vi "String length.vi"() -> ()   [LabVIEW 2020]
panel:
  out "Batch Length":i32
  out "Actual Bitrate kHz 2":i32=1000
  out "dup Cheetah Handle":i32
  out "Total Shifted Out":i32
  out "Actual Bitrate kHz":i32=1000
  out "error out":errorcluster
  in  "Rds per Sec":dbl=2000.0 max=2000000000.0
  out "SDO":u64[](array[numeric]) format="%x"
  in  "SCLK (kHz)":i32=2000 min=0
  out "Cheetah Handle":i32
  out "if false":string
  out "Result of comparission":string
  out "Length in bytes":i32
  out "SDI":u64[](array[numeric]) format="%.0x"
  out "Array":string[](array[string])
  in  "String":string
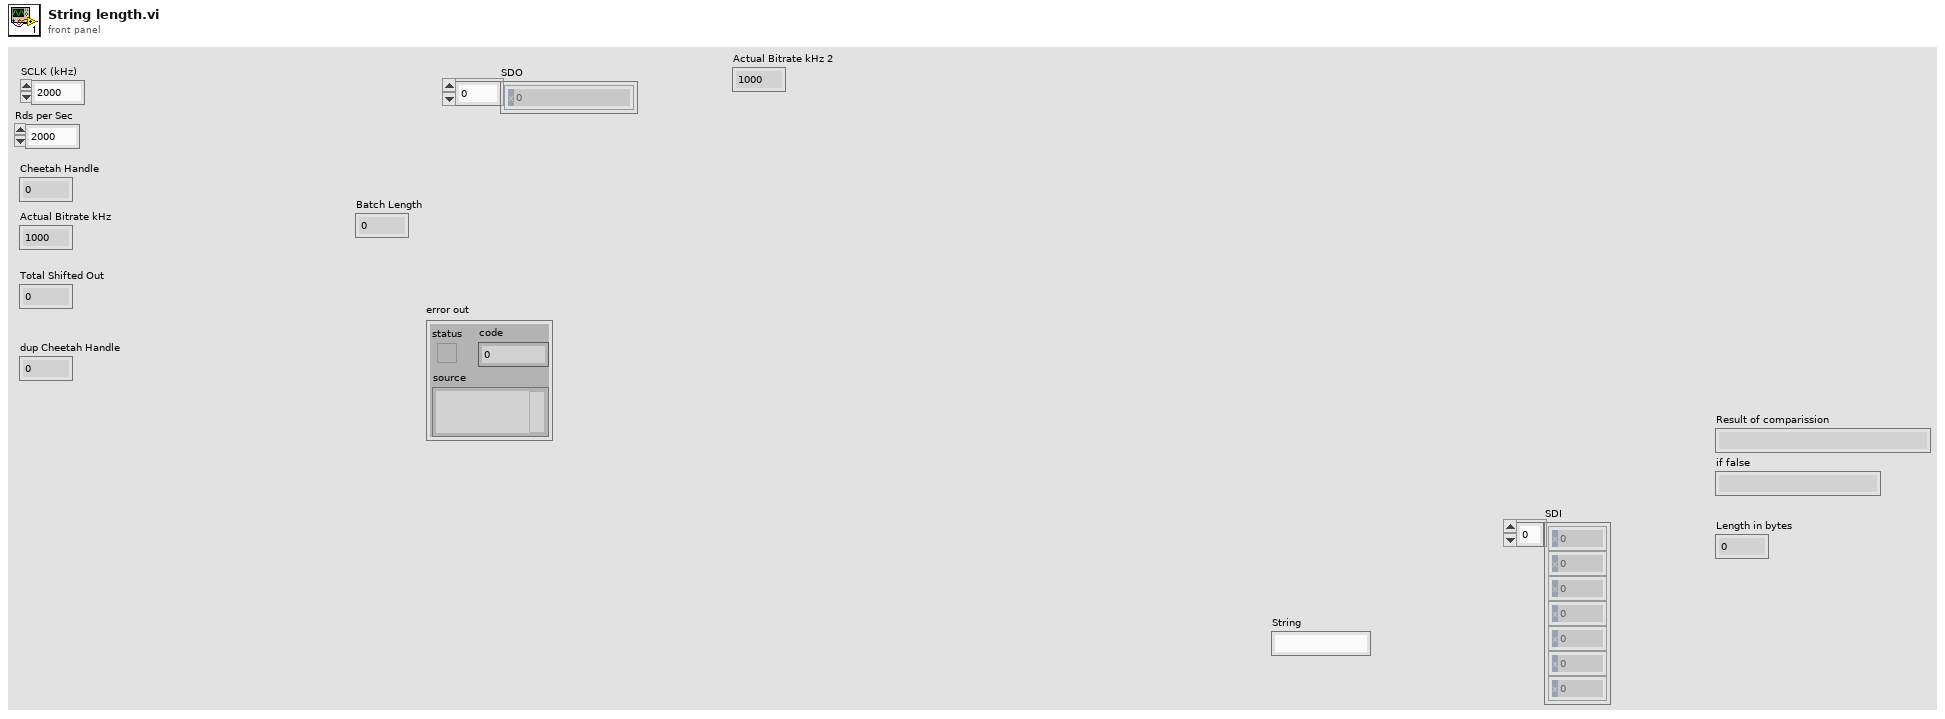
[diagram p1: front panel]
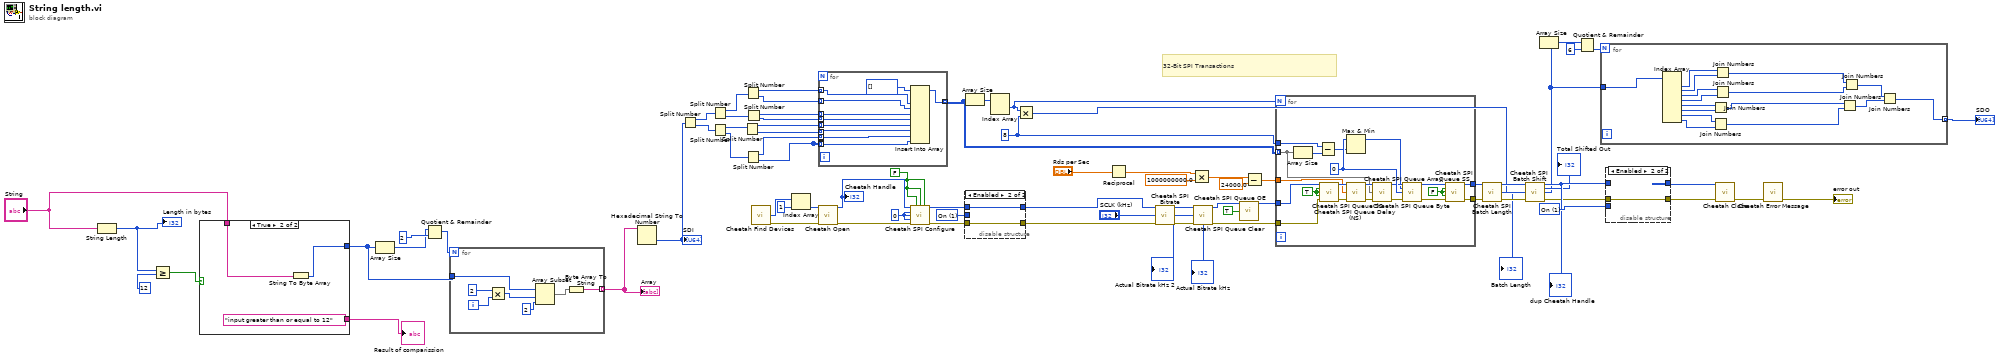
[diagram p0: block diagram]
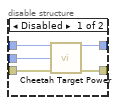
[diagram p2: hidden frame]
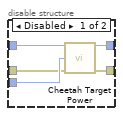
[diagram p3: hidden frame]
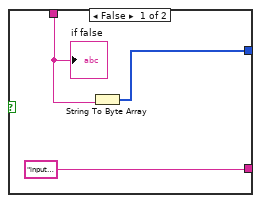
[diagram p4: hidden frame]
diagram:
  w20 = 8 ("y")
  w45 = u16 1 items=["Off", "On", "Query"] ("Requested Configuration (2: Query)")
  w46 = u16 1 items=["Off", "On", "Query"] ("Requested Configuration (2: Query)")
  w61 = FALSE
  w63 = 0
  # "32-Bit SPI Transactions"
  n1 = String Length(string="String") -> (length=w68:i32)
  "Length in bytes" <- w68
  n2 = Greater Or Equal?(x=w68, y=12) -> (x >= y?=w72:bool)
  n3 = case shown="True" w72 {
    tunnel: [w76 w81] -> w71
    tunnel: "String" -> [w77 w80]
    tunnel: ["input less than 12" "input greater than or equal to 12"] -> w69
    frame False {
      n4 = String To Byte Array(string=w77) -> (unsigned byte array=w76:u8[])
      "if false" <- w77
    }
    frame True {
      n5 = String To Byte Array(string=w80) -> (unsigned byte array=w81:u8[])
    }
  }
  "Result of comparission" <- w69
  n6 = Array Size(array=w71) -> (size(s)=w66:i32)
  n7 = Quotient & Remainder(x=w66, y=2) -> (floor(x/y)=w75:i32)  [unwired: 1 out]
  n8 = for {
    N: w75 -> [_]
    tunnel: w71 -> [w88]
    tunnel: [w85] -> w74 mode=indexing
    i -> [w83]
    n9 = Multiply(x=2 ("y"), y=w83) -> (x*y=w87:i32)
    n10 = Array Subset(array=w88, index=w87, length=2) -> (w84:u8[])
    n11 = Byte Array To String(unsigned byte array=w84) -> (string=w85:string)
  }
  "Array" <- w74
  n12 = Hexadecimal String To Number(string=w74) -> (number=w1:u32[])  [unwired: 2 in, 1 out]
  "SDI" <- w1
  n13 = Split Number(x=w1) -> (hi(x)=w31:u16[], lo(x)=w30:u16[])
  n14 = Split Number(x=w31) -> (hi(x)=w8:u8[], lo(x)=w7:u8[])
  n15 = Split Number(x=w30) -> (hi(x)=w10:u8[], lo(x)=w9:u8[])
  n16 = Split Number(x=w10) -> (hi(x)=w14:u8[], lo(x)=w13:u8[])
  n17 = Split Number(x=w8) -> (hi(x)=w6:u8[], lo(x)=w5:u8[])
  n18 = Split Number(x=w9) -> (hi(x)=w12:u8[], lo(x)=w11:u8[])
  n19 = Split Number(x=w7) -> (hi(x)=w4:u8[], lo(x)=w3:u8[])
  n20 = call <instrlib>:"Cheetah Find Devices.vi"() -> ("Ports"=w64:u16[], "error out"=w60:errorcluster)  [unwired: 13 in, 1 out]
  n21 = Index Array(array=w64, index=1) -> (element=w52:u16)
  n22 = for {
    tunnel: w14 -> [w98] mode=indexing
    tunnel: [w97] -> w29 mode=indexing
    tunnel: w12 -> [w95] mode=indexing
    tunnel: w11 -> [_] mode=indexing
    tunnel: w11 -> [w94] mode=indexing
    tunnel: w13 -> [w93] mode=indexing
    tunnel: w6 -> [w92] mode=indexing
    tunnel: w5 -> [w91] mode=indexing
    tunnel: w4 -> [w90] mode=indexing
    tunnel: w3 -> [w89] mode=indexing
    n23 = Insert Into Array(array=u8[] [], new element #1=w92, new element #2=w91, new element #3=w90, new element #4=w89, new element #5=w98, new element #6=w93, new element #7=w95, new element #8=w94) -> (w97:u8[])  [unwired: 1 in]
  }
  n24 = call <instrlib>:"Cheetah Open.vi"("Port Number (0)"=w52, "error in (no error)"=w60) -> ("Cheetah Handle"=w57:i32, "error out"=w59:errorcluster)  [unwired: 12 in]
  "Cheetah Handle" <- w57
  n25 = call <instrlib>:"Cheetah SPI Configure.vi"("Cheetah Handle"=w57, "SS0 Active High? (False)"=w61, "SS1 Active High? (False)"=w61, "SS2 Active High? (False)"=w61, "Polarity (0: Rising/Falling)"=w63, "Phase (0: Sample/Setup)"=w63, "Bitorder (0: MSB)"=w63, "error in (no error)"=w59) -> ("dup Cheetah Handle"=w56:i32, "error out"=w58:errorcluster)  [unwired: 6 in]
  n26 = disable-structure shown="Enabled" {
    disable-tunnel: w58 -> [w103 w104]
    disable-tunnel: w56 -> [w102 w105]
    disable-tunnel: [w101 w104] -> w55
    disable-tunnel: [w100 w105] -> w53
    disable-tunnel: w45 -> [w99 _]
    frame Disabled {
      n27 = call <instrlib>:"Cheetah Target Power.vi"("Cheetah Handle"=w102, "Requested Configuration (2: Query)"=w99, "error in (no error)"=w103) -> ("dup Cheetah Handle"=w100:i32, "error out"=w101:errorcluster)  [unwired: 10 in, 1 out]
    }
    frame Enabled {
    }
  }
  n28 = Array Size(array=w29) -> (size(s)=w44:i32[])
  n29 = Index Array(array=w44) -> (element #1=w16:i32)  [unwired: 2 in, 1 out]
  n30 = Multiply(x=w16, y=w20) -> (x*y=w15:i32)
  n31 = Reciprocal(x="Rds per Sec") -> (1/x=w22:dbl)
  n32 = call <instrlib>:"Cheetah SPI Bitrate.vi"("Cheetah Handle"=w53, "Requested Bitrate kHz (1000)"="SCLK (kHz)", "error in (no error)"=w55) -> ("dup Cheetah Handle"=w51:i32, "Actual Bitrate kHz"=→"Actual Bitrate kHz" →"Actual Bitrate kHz 2":i32, "error out"=w50:errorcluster)  [unwired: 10 in]
  n33 = Multiply(x=w22, y=1000000000.0) -> (x*y=w25:dbl)
  n34 = call <instrlib>:"Cheetah SPI Queue Clear.vi"("Cheetah Handle"=w51, "error in (no error)"=w50) -> ("dup Cheetah Handle"=w43:i32, "error out"=w62:errorcluster)  [unwired: 12 in]
  n35 = call <instrlib>:"Cheetah SPI Queue OE.vi"("Cheetah Handle"=w43, "Output Enable (on)"=TRUE) -> ("dup Cheetah Handle"=w42:i32)  [unwired: 12 in, 1 out]
  n36 = Subtract(x=w25, y=24000.0) -> (x-y=w23:dbl)
  n37 = for {
    N: w16 -> [_]
    tunnel: w62 -> [w112]
    tunnel: w42 -> [w113]
    tunnel: w29 -> [w114] mode=indexing
    tunnel: [w111] -> w40
    tunnel: [w110] -> w39
    tunnel: w23 -> [w107]
    tunnel: w20 -> [w108]
    w118 = FALSE
    w121 = 0
    w109 = TRUE
    n38 = Array Size(array=w114) -> (size(s)=w115:i32)
    n39 = Subtract(x=w108, y=w115) -> (x-y=w119:i32)
    n40 = call <instrlib>:"Cheetah SPI Queue SS.vi"("Cheetah Handle"=w113, "SS0 Assert? (True)"=w109, "SS1 Assert? (True)"=w109, "SS2 Assert? (True)"=w109, "error in (no error)"=w112) -> ("dup Cheetah Handle"=w126:i32, "error out"=w125:errorcluster)  [unwired: 9 in]
    n41 = Max & Min(x=w121, y=w119) -> (max(x,y)=w106:i32)  [unwired: 1 out]
    n42 = call <instrlib>:"Cheetah SPI Queue Delay (NS).vi"("Cheetah Handle"=w126, "Delay NS (1000)"=w107, "error in (no error)"=w125) -> ("dup Cheetah Handle"=w124:i32, "error out"=w123:errorcluster)  [unwired: 10 in, 1 out]
    n43 = call <instrlib>:"Cheetah SPI Queue Array.vi"("Cheetah Handle"=w124, "Data Out (none)"=w114, "error in (no error)"=w123) -> ("dup Cheetah Handle"=w120:i32, "error out"=w122:errorcluster)  [unwired: 11 in]
    n44 = call <instrlib>:"Cheetah SPI Queue Byte.vi"("Cheetah Handle"=w120, "Byte Count (1)"=w106, "Byte Value (0x00)"=w121, "error in (no error)"=w122) -> ("dup Cheetah Handle"=w117:i32, "error out"=w116:errorcluster)  [unwired: 10 in]
    n45 = call <instrlib>:"Cheetah SPI Queue SS.vi"("Cheetah Handle"=w117, "SS0 Assert? (True)"=w118, "SS1 Assert? (True)"=w118, "SS2 Assert? (True)"=w118, "error in (no error)"=w116) -> ("dup Cheetah Handle"=w110:i32, "error out"=w111:errorcluster)  [unwired: 9 in]
  }
  n46 = call <instrlib>:"Cheetah SPI Batch Length.vi"("Cheetah Handle"=w39, "error in (no error)"=w40) -> ("dup Cheetah Handle"=w38:i32, "Batch Length"=→"Batch Length":i32, "error out"=w37:errorcluster)  [unwired: 11 in]
  n47 = call <instrlib>:"Cheetah SPI Batch Shift.vi"("Cheetah Handle"=w38, "Max Bytes to Retrieve (256)"=w15, "error in (no error)"=w37) -> ("dup Cheetah Handle"=w36:i32, "Total Shifted Out"=→"Total Shifted Out":i32, "Data In"=w17:u8[], "error out"=w28:errorcluster)  [unwired: 9 in]
  "dup Cheetah Handle" <- w36
  n48 = Array Size(array=w17) -> (size(s)=w35:i32)
  n49 = Quotient & Remainder(x=w35, y=6) -> (floor(x/y)=w33:i32)  [unwired: 1 out]
  n50 = for {
    N: w33 -> [_]
    tunnel: w17 -> [w141]
    tunnel: [w140] -> w32 mode=indexing
    n51 = Index Array(array=w141) -> (element #1=w130:u8, element #2=w129:u8, element #3=w128:u8, element #4=w127:u8, element #5=w139:u8, element #6=w138:u8, element #7=w137:u8, element #8=w136:u8)  [unwired: 8 in]
    n52 = Join Numbers(hi=w139, lo=w138) -> ((hi.lo)=w135:u16)
    n53 = Join Numbers(hi=w137, lo=w136) -> ((hi.lo)=w134:u16)
    n54 = Join Numbers(hi=w130, lo=w129) -> ((hi.lo)=w133:u16)
    n55 = Join Numbers(hi=w128, lo=w127) -> ((hi.lo)=w132:u16)
    n56 = Join Numbers(hi=w135, lo=w134) -> ((hi.lo)=w142:u32)
    n57 = Join Numbers(hi=w133, lo=w132) -> ((hi.lo)=w131:u32)
    n58 = Join Numbers(hi=w131, lo=w142) -> ((hi.lo)=w140:u64)
  }
  "SDO" <- w32
  n59 = disable-structure shown="Enabled" {
    disable-tunnel: [w147 _] -> w49
    disable-tunnel: [w146 w148] -> w48
    disable-tunnel: w46 -> [w145 _]
    disable-tunnel: w36 -> [w144 _]
    disable-tunnel: w28 -> [w143 w148]
    frame Disabled {
      n60 = call <instrlib>:"Cheetah Target Power.vi"("Cheetah Handle"=w144, "Requested Configuration (2: Query)"=w145, "error in (no error)"=w143) -> ("dup Cheetah Handle"=w147:i32, "error out"=w146:errorcluster)  [unwired: 10 in, 1 out]
    }
    frame Enabled {
    }
  }
  n61 = call <instrlib>:"Cheetah Close.vi"("Cheetah Handle"=w49, "error in (no error)"=w48) -> ("error out"=w47:errorcluster)  [unwired: 12 in, 1 out]
  n62 = call <instrlib>:"Cheetah Error Message.vi"("error in (no error)"=w47) -> ("error out"=→"error out":errorcluster)  [unwired: 10 in, 4 out]
